vi "FitParametersRAW2Pixel.vi"(8 "Pixel Size":cluster{"X Step":sgl, "Y Step":sgl}={"X Step"=5.2, "Y Step"=5.2} {"Y Step" format="%.2f"; "X Step" format="%.2f"}, 9 "Subsampling":u16=16, 10 "ROI Offset":i32[](array[numeric]), 11 "Best Fits In":dbl[](array[numeric])) -> (2 "Fits metric":T1, 3 "Fits Pixel":dbl[](array[numeric]))   [LabVIEW 2015]
panel:
  # "x"
  # "µm"
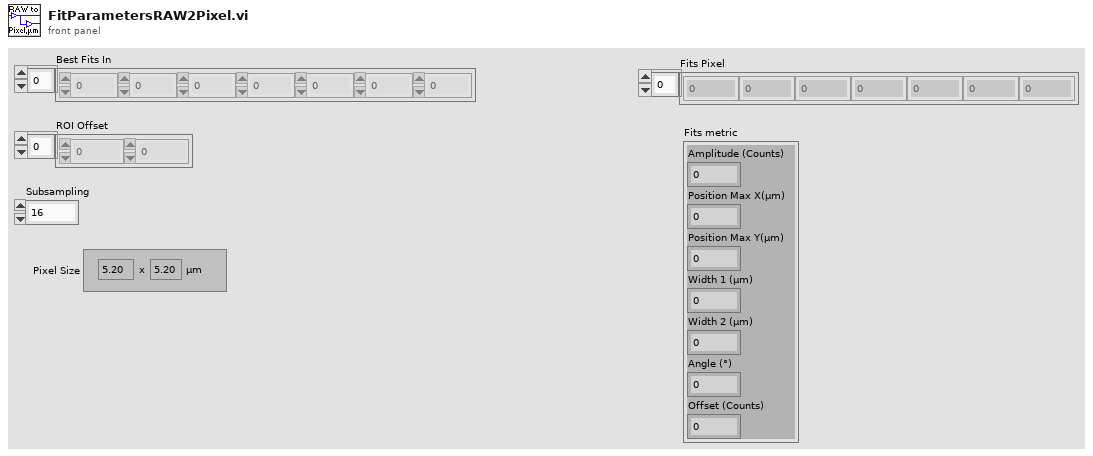
[diagram p1: front panel]
types:
  T1 = cluster{"Amplitude (Counts)":dbl, "Position Max X(µm)":dbl, "Position Max Y(µm)":dbl, "Width 1 (µm)":dbl, "Width 2 (µm)":dbl, "Angle (°)":dbl, "Offset (Counts)":dbl}
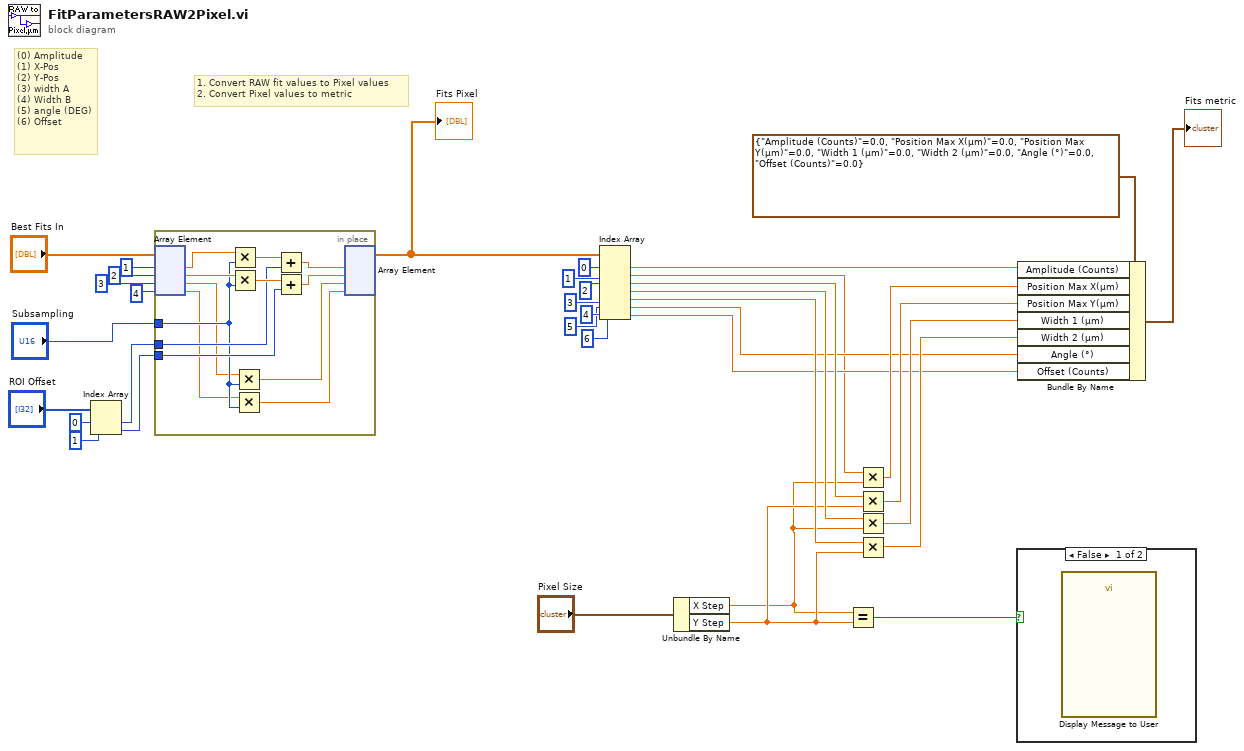
[diagram p0: block diagram]
diagram:
  # "1. Convert RAW fit values to Pixel values\n2. Convert Pixel values to metric"
  # "(0) Amplitude\n(1) X-Pos\n(2) Y-Pos\n(3) width A\n(4) Width B\n(5) angle (DEG)\n(6) Offset"
  n1 = Index Array(array="ROI Offset", index #1=0 ("index"), index #2=1 ("index")) -> (element #1=w3:i32, element #2=w1:i32)
  n2 = in-place {
    in-place-border: "Subsampling" -> [w41]
    in-place-border: w3 -> [w45]
    in-place-border: w1 -> [w44]
    n3 = in-place-array #1("Best Fits In", 1 ("index"), 2 ("index"), 3 ("index"), 4 ("index")) -> (w49:dbl, w48:dbl, w40:dbl, w39:dbl)
    n4 = Multiply(x=w49, y=w41) -> (x*y=w47:dbl)
    n5 = Multiply(x=w48, y=w41) -> (x*y=w46:dbl)
    n6 = Multiply(x=w40, y=w41) -> (x*y=w38:dbl)
    n7 = Multiply(x=w39, y=w41) -> (x*y=w37:dbl)
    n8 = Add(x=w47, y=w45) -> (x+y=w43:dbl)
    n9 = Add(x=w46, y=w44) -> (x+y=w42:dbl)
    n10 = in-place-array #1(w43, w42, w38, w37) -> (w4:dbl[])  [unwired: 4 out]
  }
  "Fits Pixel" <- w4
  n11 = Index Array(array=w4, index #1=0 ("index"), index #2=1 ("index"), index #3=2 ("index"), index #4=3 ("index"), index #5=4 ("index"), index #6=5 ("index"), index #7=6 ("index")) -> (element #1=w12:dbl, element #2=w2:dbl, element #3=w23:dbl, element #4=w24:dbl, element #5=w25:dbl, element #6=w13:dbl, element #7=w14:dbl)
  n12 = Unbundle By Name("Pixel Size") -> ("X Step"=w21:sgl, "Y Step"=w22:sgl)
  n13 = Equal?(x=w21, y=w22) -> (x = y?=w16:bool)
  n14 = Multiply(x=w2, y=w21) -> (x*y=w17:dbl)
  n15 = Multiply(x=w23, y=w22) -> (x*y=w18:dbl)
  n16 = Multiply(x=w24, y=w21) -> (x*y=w19:dbl)
  n17 = Multiply(x=w25, y=w22) -> (x*y=w20:dbl)
  n18 = case shown="False" w16 {
    frame False {
      n19 = call "Display Message to User"() -> ()  [unwired: 10 in, 2 out]
    }
    frame True {
    }
  }
  n20 = Bundle By Name(cluster=T1 {"Amplitude (Counts)"=0.0, "Position Max X(µm)"=0.0, "Position Max Y(µm)"=0.0, "Width 1 (µm)"=0.0, "Width 2 (µm)"=0.0, "Angle (°)"=0.0, "Offset (Counts)"=0.0} ("input cluster"), "Amplitude (Counts)"=w12, "Position Max X(µm)"=w17, "Position Max Y(µm)"=w18, "Width 1 (µm)"=w19, "Width 2 (µm)"=w20, "Angle (°)"=w13, "Offset (Counts)"=w14) -> (→"Fits metric":T1)
